vi "data_generation.vi"(0 "X Size":i32=8, 1 "slope":i16=10, 3 "scan range (um)":dbl=5.0, 4 "AmplitudeX":dbl=1.0, 5 "AmplitudeY":dbl=1.0, 6 "dwell time":i16=10, 7 "come back":i32, 8 "calibration":dbl=5.0, 9 "multicolor":dbl=5.0, 10 "zero point":dbl, 12 "first":dbl=0.5, 13 "Y size":i32=8, 15 "AmplitudeC":dbl=1.0, 17 "step size (um)":dbl=0.05, 18 "Samples per spot":i32=4, 19 "zero point 2":dbl) -> (2 "Output Graph":waveform(dbl)[](graph), 11 "DO":dbl[](array[numeric])=[0.0, 0.0, 0.0, 0.0, 0.0, 0.0, 0.0, 0.0, 1.0, 1.0, 1.0, 1.0, 1.0, 1.0, 1.0, 1.0, 2.0, 2.0, 2.0, 2.0, 2.0, 2.0, 2.0, 2.0, 3.0, 3.0, 3.0, 3.0, 3.0, 3.0, 3.0, 3.0, 4.0, 4.0, 4.0, 4.0, 4.0, 4.0, 4.0, 4.0, 5.0, 5.0, 5.0, 5.0, 5.0, 5.0, 5.0, 5.0, 6.0, 6.0, 6.0, 6.0, 6.0, 6.0, 6.0, 6.0, 7.0, 7.0, 7.0, 7.0, 7.0, 7.0, 7.0, 7.0, 7.0, 7.0, 7.0, 7.0, 7.0, 7.0, 7.0, 7.0, 6.0, 6.0, 6.0, 6.0, 6.0, 6.0, 6.0, 6.0, 5.0, 5.0, 5.0, 5.0, 5.0, 5.0, 5.0, 5.0, 4.0, 4.0, 4.0, 4.0, 4.0, 4.0, 4.0, 4.0, 3.0, 3.0, 3.0, 3.0, 3.0, 3.0, 3.0, 3.0, 2.0, 2.0, 2.0, 2.0, 2.0, 2.0, 2.0, 2.0, 1.0, 1.0, 1.0, 1.0, 1.0, 1.0, 1.0, 1.0, 0.0, 0.0, 0.0, 0.0, 0.0, 0.0, 0.0, 0.0], 14 "XY Scan":waveform(dbl)[](array[waveform])=[{"t0"=timestamp(3264022747.299 s since 1904-01-01), "dt"=0.015625, "Y"=[-1.0, -0.7142857142857143, -0.4285714285714286, -0.1428571428571429, 0.1428571428571428, 0.4285714285714286, 0.7142857142857142, 1.0, 1.0, 0.7142857142857142, 0.4285714285714286, 0.1428571428571428, -0.1428571428571429, -0.4285714285714286, -0.7142857142857143, -1.0, -1.0, -0.7142857142857143, -0.4285714285714286, -0.1428571428571429, 0.1428571428571428, 0.4285714285714286, 0.7142857142857142, 1.0, 1.0, 0.7142857142857142, 0.4285714285714286, 0.1428571428571428, -0.1428571428571429, -0.4285714285714286, -0.7142857142857143, -1.0, -1.0, -0.7142857142857143, -0.4285714285714286, -0.1428571428571429, 0.1428571428571428, 0.4285714285714286, 0.7142857142857142, 1.0, 1.0, 0.7142857142857142, 0.4285714285714286, 0.1428571428571428, -0.1428571428571429, -0.4285714285714286, -0.7142857142857143, -1.0, -1.0, -0.7142857142857143, -0.4285714285714286, -0.1428571428571429, 0.1428571428571428, 0.4285714285714286, 0.7142857142857142, 1.0, 1.0, 0.7142857142857142, 0.4285714285714286, 0.1428571428571428, -0.1428571428571429, -0.4285714285714286, -0.7142857142857143, -1.0, -1.0, -0.7142857142857143, -0.4285714285714286, -0.1428571428571429, 0.1428571428571428, 0.4285714285714286, 0.7142857142857142, 1.0, 1.0, 0.7142857142857142, 0.4285714285714286, 0.1428571428571428, -0.1428571428571429, -0.4285714285714286, -0.7142857142857143, -1.0, -1.0, -0.7142857142857143, -0.4285714285714286, -0.1428571428571429, 0.1428571428571428, 0.4285714285714286, 0.7142857142857142, 1.0, 1.0, 0.7142857142857142, 0.4285714285714286, 0.1428571428571428, -0.1428571428571429, -0.4285714285714286, -0.7142857142857143, -1.0, -1.0, -0.7142857142857143, -0.4285714285714286, -0.1428571428571429, 0.1428571428571428, 0.4285714285714286, 0.7142857142857142, 1.0, 1.0, 0.7142857142857142, 0.4285714285714286, 0.1428571428571428, -0.1428571428571429, -0.4285714285714286, -0.7142857142857143, -1.0, -1.0, -0.7142857142857143, -0.4285714285714286, -0.1428571428571429, 0.1428571428571428, 0.4285714285714286, 0.7142857142857142, 1.0, 1.0, 0.7142857142857142, 0.4285714285714286, 0.1428571428571428, -0.1428571428571429, -0.4285714285714286, -0.7142857142857143, -1.0]}, {"t0"=timestamp(3264022747.299 s since 1904-01-01), "dt"=0.015625, "Y"=[-1.0, -1.0, -1.0, -1.0, -1.0, -1.0, -1.0, -1.0, -0.7142857142857143, -0.7142857142857143, -0.7142857142857143, -0.7142857142857143, -0.7142857142857143, -0.7142857142857143, -0.7142857142857143, -0.7142857142857143, -0.4285714285714286, -0.4285714285714286, -0.4285714285714286, -0.4285714285714286, -0.4285714285714286, -0.4285714285714286, -0.4285714285714286, -0.4285714285714286, -0.1428571428571429, -0.1428571428571429, -0.1428571428571429, -0.1428571428571429, -0.1428571428571429, -0.1428571428571429, -0.1428571428571429, -0.1428571428571429, 0.1428571428571428, 0.1428571428571428, 0.1428571428571428, 0.1428571428571428, 0.1428571428571428, 0.1428571428571428, 0.1428571428571428, 0.1428571428571428, 0.4285714285714286, 0.4285714285714286, 0.4285714285714286, 0.4285714285714286, 0.4285714285714286, 0.4285714285714286, 0.4285714285714286, 0.4285714285714286, 0.7142857142857142, 0.7142857142857142, 0.7142857142857142, 0.7142857142857142, 0.7142857142857142, 0.7142857142857142, 0.7142857142857142, 0.7142857142857142, 1.0, 1.0, 1.0, 1.0, 1.0, 1.0, 1.0, 1.0, 1.0, 1.0, 1.0, 1.0, 1.0, 1.0, 1.0, 1.0, 0.7142857142857142, 0.7142857142857142, 0.7142857142857142, 0.7142857142857142, 0.7142857142857142, 0.7142857142857142, 0.7142857142857142, 0.7142857142857142, 0.4285714285714286, 0.4285714285714286, 0.4285714285714286, 0.4285714285714286, 0.4285714285714286, 0.4285714285714286, 0.4285714285714286, 0.4285714285714286, 0.1428571428571428, 0.1428571428571428, 0.1428571428571428, 0.1428571428571428, 0.1428571428571428, 0.1428571428571428, 0.1428571428571428, 0.1428571428571428, -0.1428571428571429, -0.1428571428571429, -0.1428571428571429, -0.1428571428571429, -0.1428571428571429, -0.1428571428571429, -0.1428571428571429, -0.1428571428571429, -0.4285714285714286, -0.4285714285714286, -0.4285714285714286, -0.4285714285714286, -0.4285714285714286, -0.4285714285714286, -0.4285714285714286, -0.4285714285714286, -0.7142857142857143, -0.7142857142857143, -0.7142857142857143, -0.7142857142857143, -0.7142857142857143, -0.7142857142857143, -0.7142857142857143, -0.7142857142857143, -1.0, -1.0, -1.0, -1.0, -1.0, -1.0, -1.0, -1.0]}])   [LabVIEW 2017]
uses:
  Instance           2 16Saved   scan_1_5 .vi
  Instance           3 16Saved   scan_1_5 .vi
  <vilib>/Analysis/3filter.llb/Zero Phase Filter (DBL).vi
  <vilib>/Analysis/NI_AALBase.lvlib
panel:
  out "AO Data":dbl[][](array[numeric])
  out "nanoZ output":dbl[](array[numeric])=[-1.0, -1.0, -1.0, -1.0, -1.0, -1.0, -1.0, -1.0, -0.7142857142857143, -0.7142857142857143, -0.7142857142857143, -0.7142857142857143, -0.7142857142857143, -0.7142857142857143, -0.7142857142857143, -0.7142857142857143, -0.4285714285714286, -0.4285714285714286, -0.4285714285714286, -0.4285714285714286, -0.4285714285714286, -0.4285714285714286, -0.4285714285714286, -0.4285714285714286, -0.1428571428571429, -0.1428571428571429, -0.1428571428571429, -0.1428571428571429, -0.1428571428571429, -0.1428571428571429, -0.1428571428571429, -0.1428571428571429, 0.1428571428571428, 0.1428571428571428, 0.1428571428571428, 0.1428571428571428, 0.1428571428571428, 0.1428571428571428, 0.1428571428571428, 0.1428571428571428, 0.4285714285714286, 0.4285714285714286, 0.4285714285714286, 0.4285714285714286, 0.4285714285714286, 0.4285714285714286, 0.4285714285714286, 0.4285714285714286, 0.7142857142857142, 0.7142857142857142, 0.7142857142857142, 0.7142857142857142, 0.7142857142857142, 0.7142857142857142, 0.7142857142857142, 0.7142857142857142, 1.0, 1.0, 1.0, 1.0, 1.0, 1.0, 1.0, 1.0, 1.0, 1.0, 1.0, 1.0, 1.0, 1.0, 1.0, 1.0, 0.7142857142857142, 0.7142857142857142, 0.7142857142857142, 0.7142857142857142, 0.7142857142857142, 0.7142857142857142, 0.7142857142857142, 0.7142857142857142, 0.4285714285714286, 0.4285714285714286, 0.4285714285714286, 0.4285714285714286, 0.4285714285714286, 0.4285714285714286, 0.4285714285714286, 0.4285714285714286, 0.1428571428571428, 0.1428571428571428, 0.1428571428571428, 0.1428571428571428, 0.1428571428571428, 0.1428571428571428, 0.1428571428571428, 0.1428571428571428, -0.1428571428571429, -0.1428571428571429, -0.1428571428571429, -0.1428571428571429, -0.1428571428571429, -0.1428571428571429, -0.1428571428571429, -0.1428571428571429, -0.4285714285714286, -0.4285714285714286, -0.4285714285714286, -0.4285714285714286, -0.4285714285714286, -0.4285714285714286, -0.4285714285714286, -0.4285714285714286, -0.7142857142857143, -0.7142857142857143, -0.7142857142857143, -0.7142857142857143, -0.7142857142857143, -0.7142857142857143, -0.7142857142857143, -0.7142857142857143, -1.0, -1.0, -1.0, -1.0, -1.0, -1.0, -1.0, -1.0]
  out "nanoZ":dbl[](array[numeric])=[0.0, 1.0, 2.0, 3.0, 4.0, 5.0, 6.0, 7.0, 7.0, 6.0, 5.0, 4.0, 3.0, 2.0, 1.0, 0.0, 0.0, 1.0, 2.0, 3.0, 4.0, 5.0, 6.0, 7.0, 7.0, 6.0, 5.0, 4.0, 3.0, 2.0, 1.0, 0.0, 0.0, 1.0, 2.0, 3.0, 4.0, 5.0, 6.0, 7.0, 7.0, 6.0, 5.0, 4.0, 3.0, 2.0, 1.0, 0.0, 0.0, 1.0, 2.0, 3.0, 4.0, 5.0, 6.0, 7.0, 7.0, 6.0, 5.0, 4.0, 3.0, 2.0, 1.0, 0.0, 0.0, 1.0, 2.0, 3.0, 4.0, 5.0, 6.0, 7.0, 7.0, 6.0, 5.0, 4.0, 3.0, 2.0, 1.0, 0.0, 0.0, 1.0, 2.0, 3.0, 4.0, 5.0, 6.0, 7.0, 7.0, 6.0, 5.0, 4.0, 3.0, 2.0, 1.0, 0.0, 0.0, 1.0, 2.0, 3.0, 4.0, 5.0, 6.0, 7.0, 7.0, 6.0, 5.0, 4.0, 3.0, 2.0, 1.0, 0.0, 0.0, 1.0, 2.0, 3.0, 4.0, 5.0, 6.0, 7.0, 7.0, 6.0, 5.0, 4.0, 3.0, 2.0, 1.0, 0.0]
  out "Trigger output":dbl[](array[numeric])=[-1.0, -1.0, -1.0, -1.0, -1.0, -1.0, -1.0, -1.0, -0.7142857142857143, -0.7142857142857143, -0.7142857142857143, -0.7142857142857143, -0.7142857142857143, -0.7142857142857143, -0.7142857142857143, -0.7142857142857143, -0.4285714285714286, -0.4285714285714286, -0.4285714285714286, -0.4285714285714286, -0.4285714285714286, -0.4285714285714286, -0.4285714285714286, -0.4285714285714286, -0.1428571428571429, -0.1428571428571429, -0.1428571428571429, -0.1428571428571429, -0.1428571428571429, -0.1428571428571429, -0.1428571428571429, -0.1428571428571429, 0.1428571428571428, 0.1428571428571428, 0.1428571428571428, 0.1428571428571428, 0.1428571428571428, 0.1428571428571428, 0.1428571428571428, 0.1428571428571428, 0.4285714285714286, 0.4285714285714286, 0.4285714285714286, 0.4285714285714286, 0.4285714285714286, 0.4285714285714286, 0.4285714285714286, 0.4285714285714286, 0.7142857142857142, 0.7142857142857142, 0.7142857142857142, 0.7142857142857142, 0.7142857142857142, 0.7142857142857142, 0.7142857142857142, 0.7142857142857142, 1.0, 1.0, 1.0, 1.0, 1.0, 1.0, 1.0, 1.0, 1.0, 1.0, 1.0, 1.0, 1.0, 1.0, 1.0, 1.0, 0.7142857142857142, 0.7142857142857142, 0.7142857142857142, 0.7142857142857142, 0.7142857142857142, 0.7142857142857142, 0.7142857142857142, 0.7142857142857142, 0.4285714285714286, 0.4285714285714286, 0.4285714285714286, 0.4285714285714286, 0.4285714285714286, 0.4285714285714286, 0.4285714285714286, 0.4285714285714286, 0.1428571428571428, 0.1428571428571428, 0.1428571428571428, 0.1428571428571428, 0.1428571428571428, 0.1428571428571428, 0.1428571428571428, 0.1428571428571428, -0.1428571428571429, -0.1428571428571429, -0.1428571428571429, -0.1428571428571429, -0.1428571428571429, -0.1428571428571429, -0.1428571428571429, -0.1428571428571429, -0.4285714285714286, -0.4285714285714286, -0.4285714285714286, -0.4285714285714286, -0.4285714285714286, -0.4285714285714286, -0.4285714285714286, -0.4285714285714286, -0.7142857142857143, -0.7142857142857143, -0.7142857142857143, -0.7142857142857143, -0.7142857142857143, -0.7142857142857143, -0.7142857142857143, -0.7142857142857143, -1.0, -1.0, -1.0, -1.0, -1.0, -1.0, -1.0, -1.0]
  out "Trigger":dbl[](array[numeric])=[0.0, 0.0, 0.0, 0.0, 0.0, 0.0, 0.0, 0.0, 1.0, 1.0, 1.0, 1.0, 1.0, 1.0, 1.0, 1.0, 2.0, 2.0, 2.0, 2.0, 2.0, 2.0, 2.0, 2.0, 3.0, 3.0, 3.0, 3.0, 3.0, 3.0, 3.0, 3.0, 4.0, 4.0, 4.0, 4.0, 4.0, 4.0, 4.0, 4.0, 5.0, 5.0, 5.0, 5.0, 5.0, 5.0, 5.0, 5.0, 6.0, 6.0, 6.0, 6.0, 6.0, 6.0, 6.0, 6.0, 7.0, 7.0, 7.0, 7.0, 7.0, 7.0, 7.0, 7.0, 7.0, 7.0, 7.0, 7.0, 7.0, 7.0, 7.0, 7.0, 6.0, 6.0, 6.0, 6.0, 6.0, 6.0, 6.0, 6.0, 5.0, 5.0, 5.0, 5.0, 5.0, 5.0, 5.0, 5.0, 4.0, 4.0, 4.0, 4.0, 4.0, 4.0, 4.0, 4.0, 3.0, 3.0, 3.0, 3.0, 3.0, 3.0, 3.0, 3.0, 2.0, 2.0, 2.0, 2.0, 2.0, 2.0, 2.0, 2.0, 1.0, 1.0, 1.0, 1.0, 1.0, 1.0, 1.0, 1.0, 0.0, 0.0, 0.0, 0.0, 0.0, 0.0, 0.0, 0.0]
  out "Waveform Graph":dynamicdata(graph)
  in  "dt":dbl=1e-05
  out "time":dbl=3264022747.299 format="%<%I:%M:%S %p\n%m/%d/%Y>T"
  out "Y output Array":dbl[](array[numeric])=[-1.0, -1.0, -1.0, -1.0, -1.0, -1.0, -1.0, -1.0, -0.7142857142857143, -0.7142857142857143, -0.7142857142857143, -0.7142857142857143, -0.7142857142857143, -0.7142857142857143, -0.7142857142857143, -0.7142857142857143, -0.4285714285714286, -0.4285714285714286, -0.4285714285714286, -0.4285714285714286, -0.4285714285714286, -0.4285714285714286, -0.4285714285714286, -0.4285714285714286, -0.1428571428571429, -0.1428571428571429, -0.1428571428571429, -0.1428571428571429, -0.1428571428571429, -0.1428571428571429, -0.1428571428571429, -0.1428571428571429, 0.1428571428571428, 0.1428571428571428, 0.1428571428571428, 0.1428571428571428, 0.1428571428571428, 0.1428571428571428, 0.1428571428571428, 0.1428571428571428, 0.4285714285714286, 0.4285714285714286, 0.4285714285714286, 0.4285714285714286, 0.4285714285714286, 0.4285714285714286, 0.4285714285714286, 0.4285714285714286, 0.7142857142857142, 0.7142857142857142, 0.7142857142857142, 0.7142857142857142, 0.7142857142857142, 0.7142857142857142, 0.7142857142857142, 0.7142857142857142, 1.0, 1.0, 1.0, 1.0, 1.0, 1.0, 1.0, 1.0, 1.0, 1.0, 1.0, 1.0, 1.0, 1.0, 1.0, 1.0, 0.7142857142857142, 0.7142857142857142, 0.7142857142857142, 0.7142857142857142, 0.7142857142857142, 0.7142857142857142, 0.7142857142857142, 0.7142857142857142, 0.4285714285714286, 0.4285714285714286, 0.4285714285714286, 0.4285714285714286, 0.4285714285714286, 0.4285714285714286, 0.4285714285714286, 0.4285714285714286, 0.1428571428571428, 0.1428571428571428, 0.1428571428571428, 0.1428571428571428, 0.1428571428571428, 0.1428571428571428, 0.1428571428571428, 0.1428571428571428, -0.1428571428571429, -0.1428571428571429, -0.1428571428571429, -0.1428571428571429, -0.1428571428571429, -0.1428571428571429, -0.1428571428571429, -0.1428571428571429, -0.4285714285714286, -0.4285714285714286, -0.4285714285714286, -0.4285714285714286, -0.4285714285714286, -0.4285714285714286, -0.4285714285714286, -0.4285714285714286, -0.7142857142857143, -0.7142857142857143, -0.7142857142857143, -0.7142857142857143, -0.7142857142857143, -0.7142857142857143, -0.7142857142857143, -0.7142857142857143, -1.0, -1.0, -1.0, -1.0, -1.0, -1.0, -1.0, -1.0]
  out "X output Array":dbl[](array[numeric])=[-1.0, -0.7142857142857143, -0.4285714285714286, -0.1428571428571429, 0.1428571428571428, 0.4285714285714286, 0.7142857142857142, 1.0, 1.0, 0.7142857142857142, 0.4285714285714286, 0.1428571428571428, -0.1428571428571429, -0.4285714285714286, -0.7142857142857143, -1.0, -1.0, -0.7142857142857143, -0.4285714285714286, -0.1428571428571429, 0.1428571428571428, 0.4285714285714286, 0.7142857142857142, 1.0, 1.0, 0.7142857142857142, 0.4285714285714286, 0.1428571428571428, -0.1428571428571429, -0.4285714285714286, -0.7142857142857143, -1.0, -1.0, -0.7142857142857143, -0.4285714285714286, -0.1428571428571429, 0.1428571428571428, 0.4285714285714286, 0.7142857142857142, 1.0, 1.0, 0.7142857142857142, 0.4285714285714286, 0.1428571428571428, -0.1428571428571429, -0.4285714285714286, -0.7142857142857143, -1.0, -1.0, -0.7142857142857143, -0.4285714285714286, -0.1428571428571429, 0.1428571428571428, 0.4285714285714286, 0.7142857142857142, 1.0, 1.0, 0.7142857142857142, 0.4285714285714286, 0.1428571428571428, -0.1428571428571429, -0.4285714285714286, -0.7142857142857143, -1.0, -1.0, -0.7142857142857143, -0.4285714285714286, -0.1428571428571429, 0.1428571428571428, 0.4285714285714286, 0.7142857142857142, 1.0, 1.0, 0.7142857142857142, 0.4285714285714286, 0.1428571428571428, -0.1428571428571429, -0.4285714285714286, -0.7142857142857143, -1.0, -1.0, -0.7142857142857143, -0.4285714285714286, -0.1428571428571429, 0.1428571428571428, 0.4285714285714286, 0.7142857142857142, 1.0, 1.0, 0.7142857142857142, 0.4285714285714286, 0.1428571428571428, -0.1428571428571429, -0.4285714285714286, -0.7142857142857143, -1.0, -1.0, -0.7142857142857143, -0.4285714285714286, -0.1428571428571429, 0.1428571428571428, 0.4285714285714286, 0.7142857142857142, 1.0, 1.0, 0.7142857142857142, 0.4285714285714286, 0.1428571428571428, -0.1428571428571429, -0.4285714285714286, -0.7142857142857143, -1.0, -1.0, -0.7142857142857143, -0.4285714285714286, -0.1428571428571429, 0.1428571428571428, 0.4285714285714286, 0.7142857142857142, 1.0, 1.0, 0.7142857142857142, 0.4285714285714286, 0.1428571428571428, -0.1428571428571429, -0.4285714285714286, -0.7142857142857143, -1.0]
  out "Y index Array":dbl[](array[numeric])=[0.0, 0.0, 0.0, 0.0, 0.0, 0.0, 0.0, 0.0, 1.0, 1.0, 1.0, 1.0, 1.0, 1.0, 1.0, 1.0, 2.0, 2.0, 2.0, 2.0, 2.0, 2.0, 2.0, 2.0, 3.0, 3.0, 3.0, 3.0, 3.0, 3.0, 3.0, 3.0, 4.0, 4.0, 4.0, 4.0, 4.0, 4.0, 4.0, 4.0, 5.0, 5.0, 5.0, 5.0, 5.0, 5.0, 5.0, 5.0, 6.0, 6.0, 6.0, 6.0, 6.0, 6.0, 6.0, 6.0, 7.0, 7.0, 7.0, 7.0, 7.0, 7.0, 7.0, 7.0, 7.0, 7.0, 7.0, 7.0, 7.0, 7.0, 7.0, 7.0, 6.0, 6.0, 6.0, 6.0, 6.0, 6.0, 6.0, 6.0, 5.0, 5.0, 5.0, 5.0, 5.0, 5.0, 5.0, 5.0, 4.0, 4.0, 4.0, 4.0, 4.0, 4.0, 4.0, 4.0, 3.0, 3.0, 3.0, 3.0, 3.0, 3.0, 3.0, 3.0, 2.0, 2.0, 2.0, 2.0, 2.0, 2.0, 2.0, 2.0, 1.0, 1.0, 1.0, 1.0, 1.0, 1.0, 1.0, 1.0, 0.0, 0.0, 0.0, 0.0, 0.0, 0.0, 0.0, 0.0]
  out "X index Array":dbl[](array[numeric])=[0.0, 1.0, 2.0, 3.0, 4.0, 5.0, 6.0, 7.0, 7.0, 6.0, 5.0, 4.0, 3.0, 2.0, 1.0, 0.0, 0.0, 1.0, 2.0, 3.0, 4.0, 5.0, 6.0, 7.0, 7.0, 6.0, 5.0, 4.0, 3.0, 2.0, 1.0, 0.0, 0.0, 1.0, 2.0, 3.0, 4.0, 5.0, 6.0, 7.0, 7.0, 6.0, 5.0, 4.0, 3.0, 2.0, 1.0, 0.0, 0.0, 1.0, 2.0, 3.0, 4.0, 5.0, 6.0, 7.0, 7.0, 6.0, 5.0, 4.0, 3.0, 2.0, 1.0, 0.0, 0.0, 1.0, 2.0, 3.0, 4.0, 5.0, 6.0, 7.0, 7.0, 6.0, 5.0, 4.0, 3.0, 2.0, 1.0, 0.0, 0.0, 1.0, 2.0, 3.0, 4.0, 5.0, 6.0, 7.0, 7.0, 6.0, 5.0, 4.0, 3.0, 2.0, 1.0, 0.0, 0.0, 1.0, 2.0, 3.0, 4.0, 5.0, 6.0, 7.0, 7.0, 6.0, 5.0, 4.0, 3.0, 2.0, 1.0, 0.0, 0.0, 1.0, 2.0, 3.0, 4.0, 5.0, 6.0, 7.0, 7.0, 6.0, 5.0, 4.0, 3.0, 2.0, 1.0, 0.0]
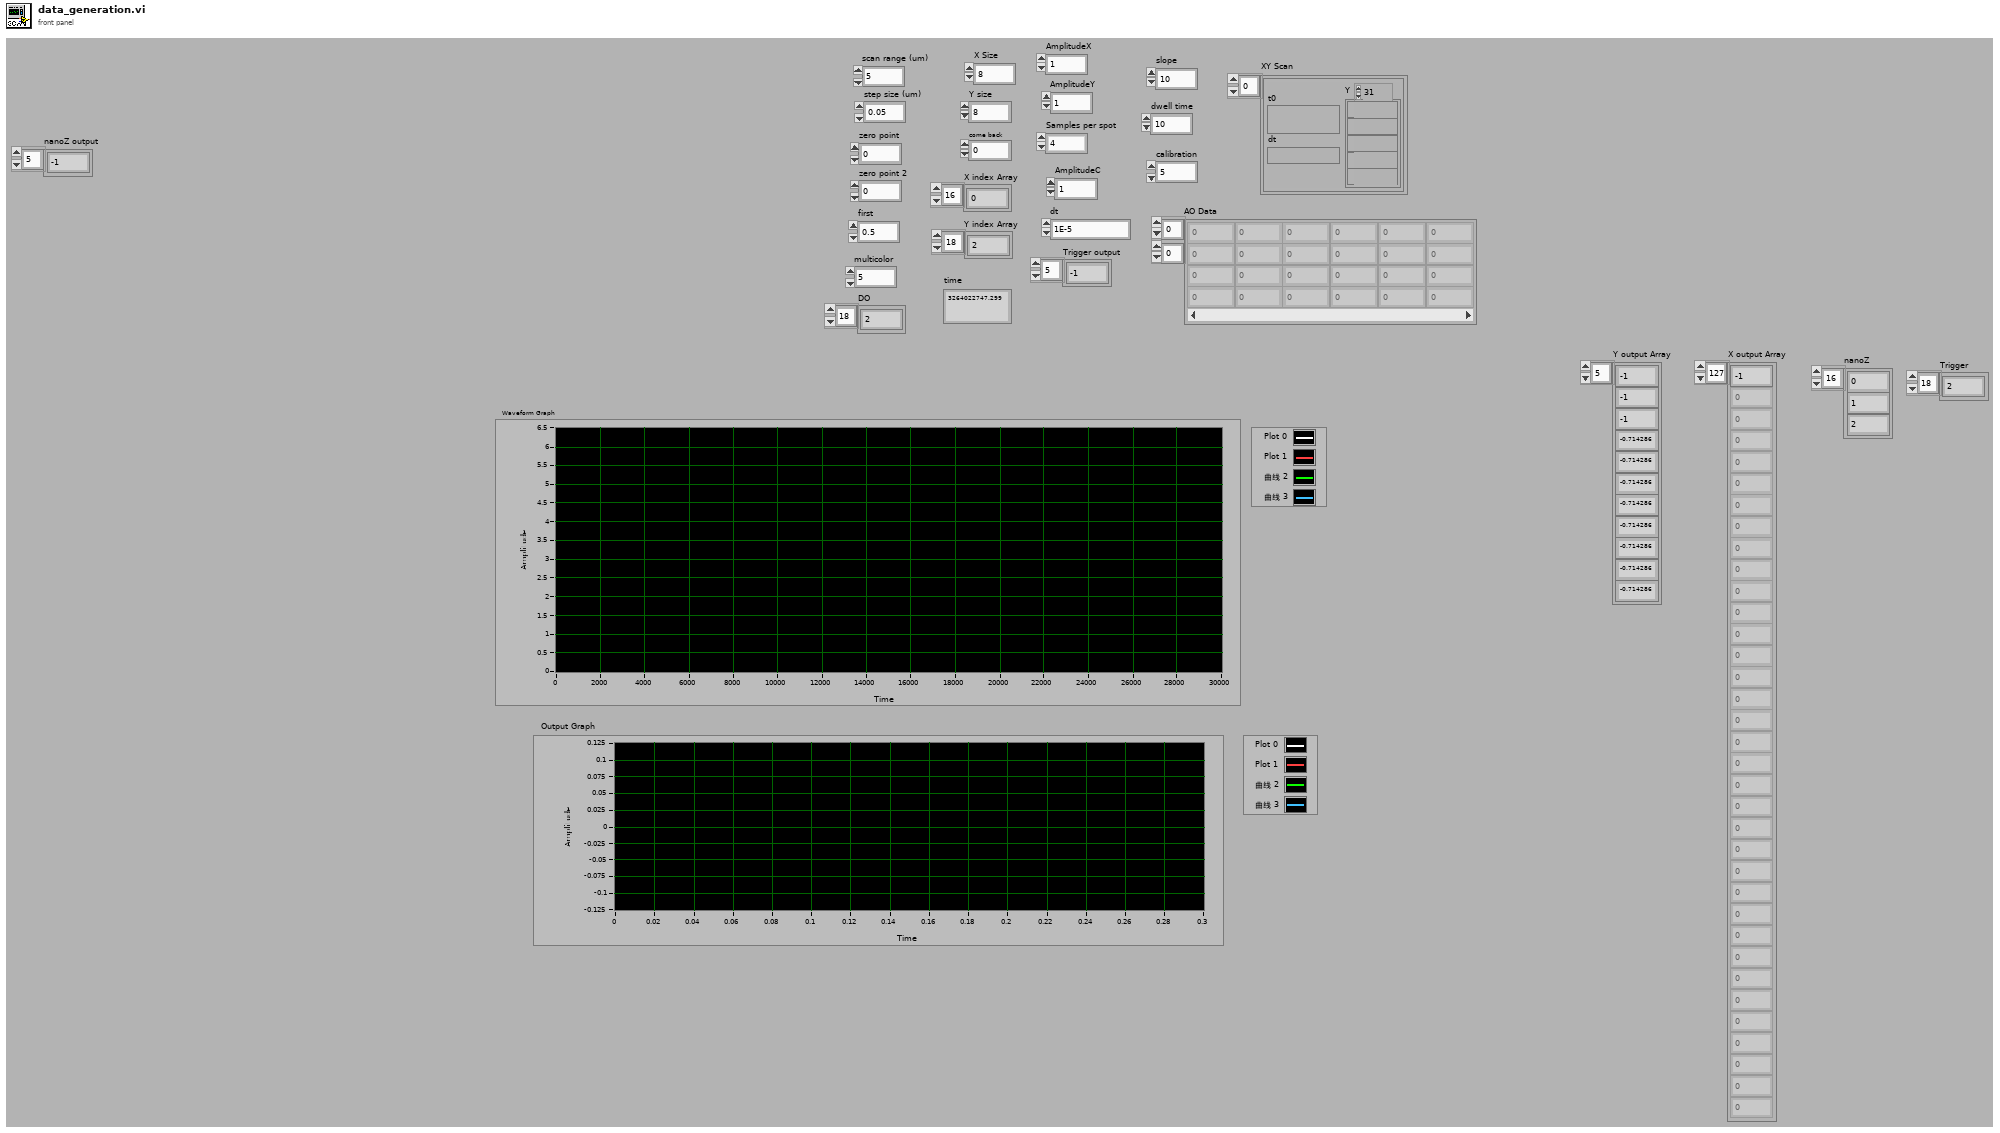
[diagram p1: front panel]
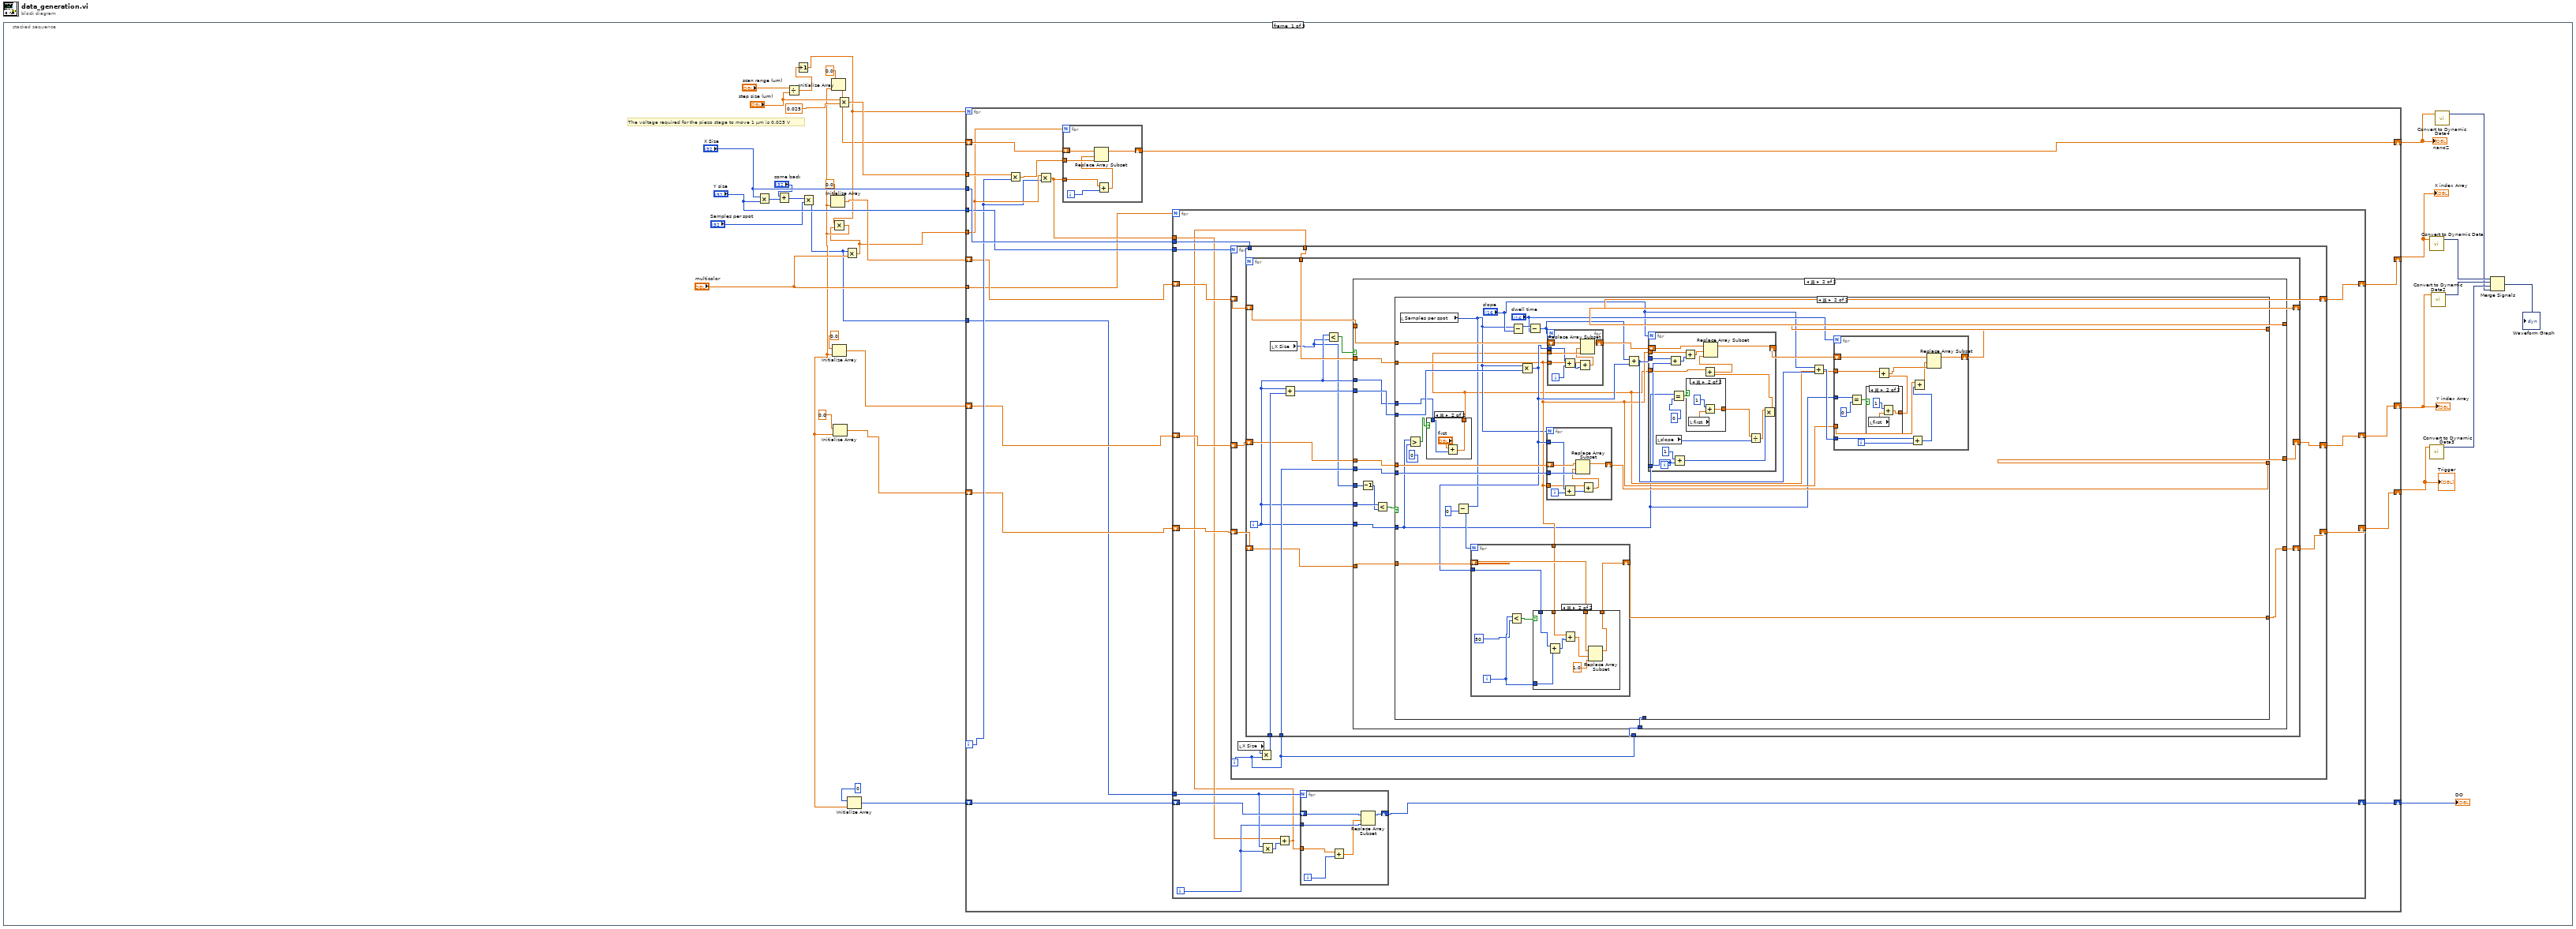
[diagram p0: block diagram]
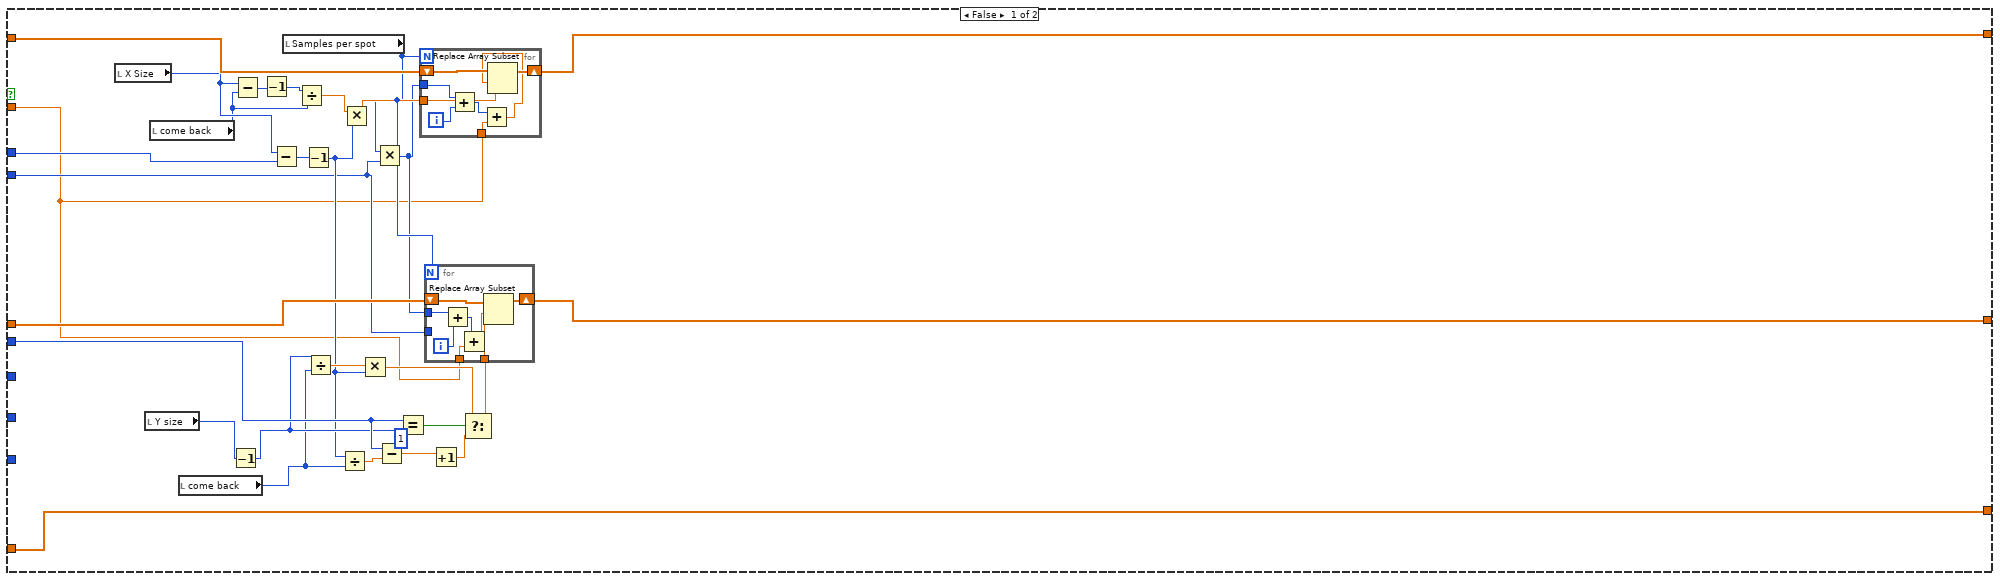
[diagram p2: hidden frame]
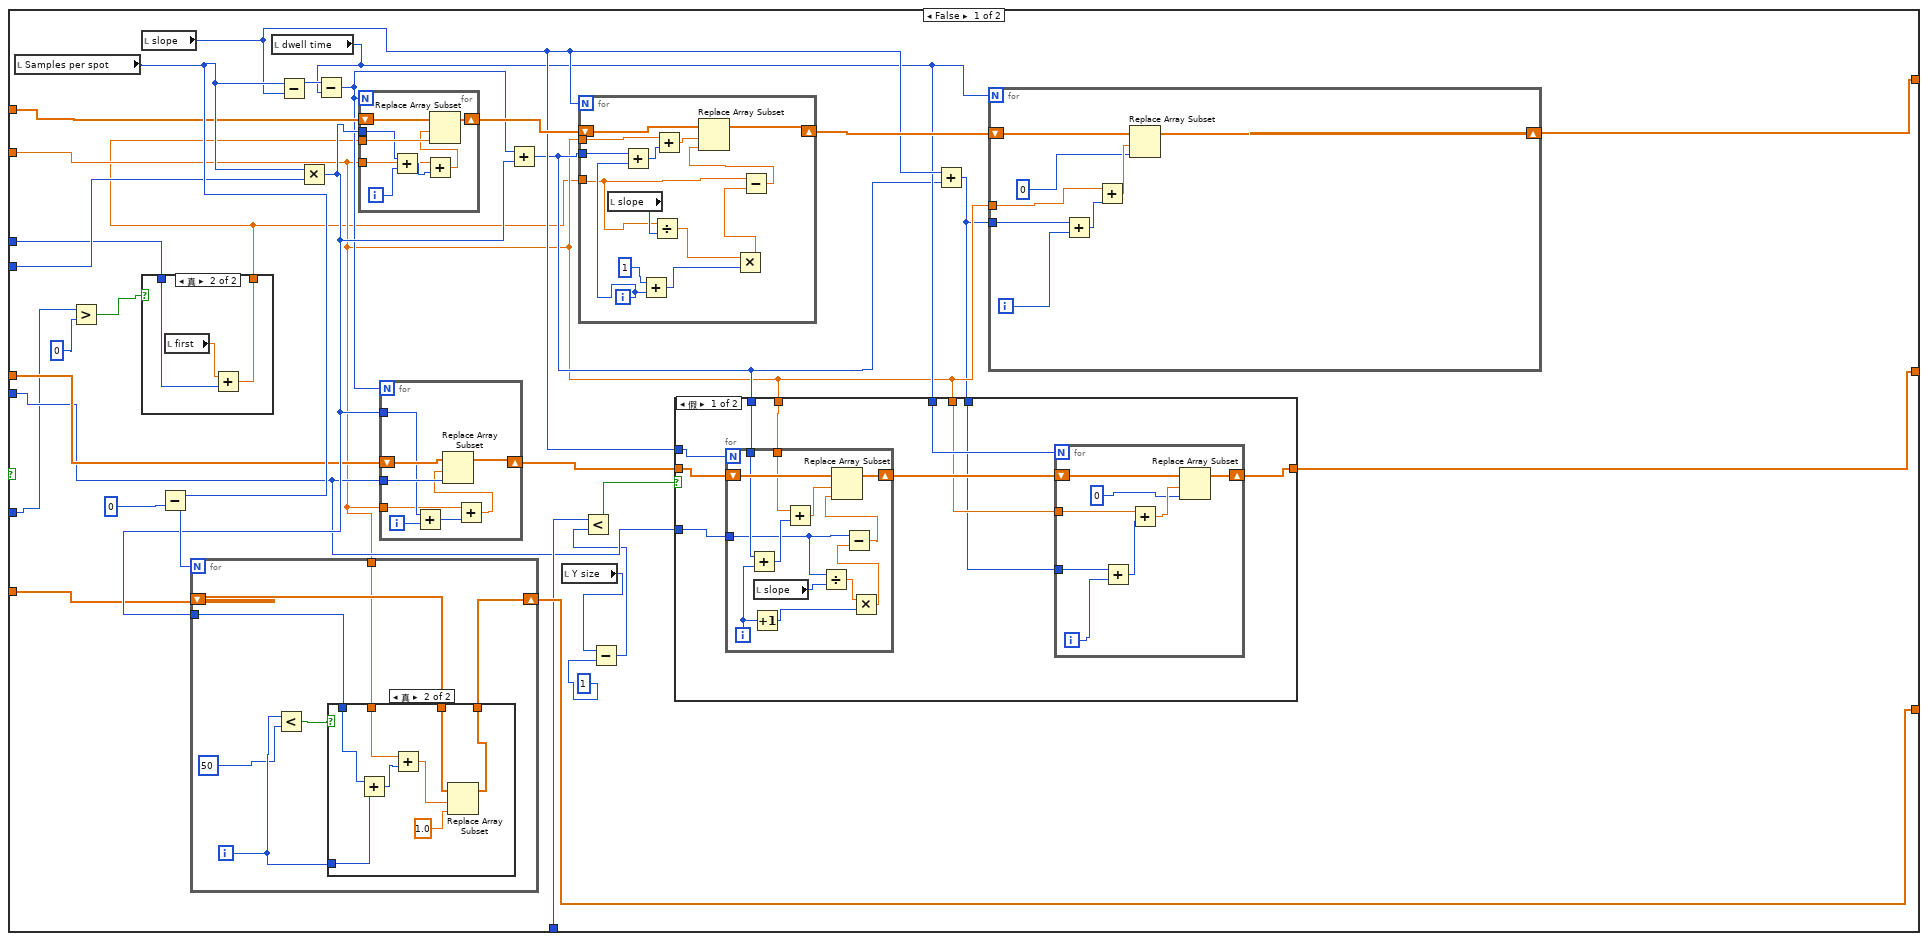
[diagram p3: hidden frame]
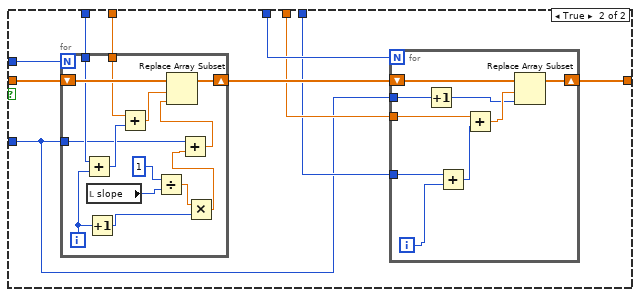
[diagram p5: hidden frame]
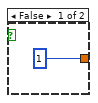
[diagram p8: hidden frame]
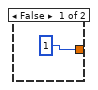
[diagram p9: hidden frame]
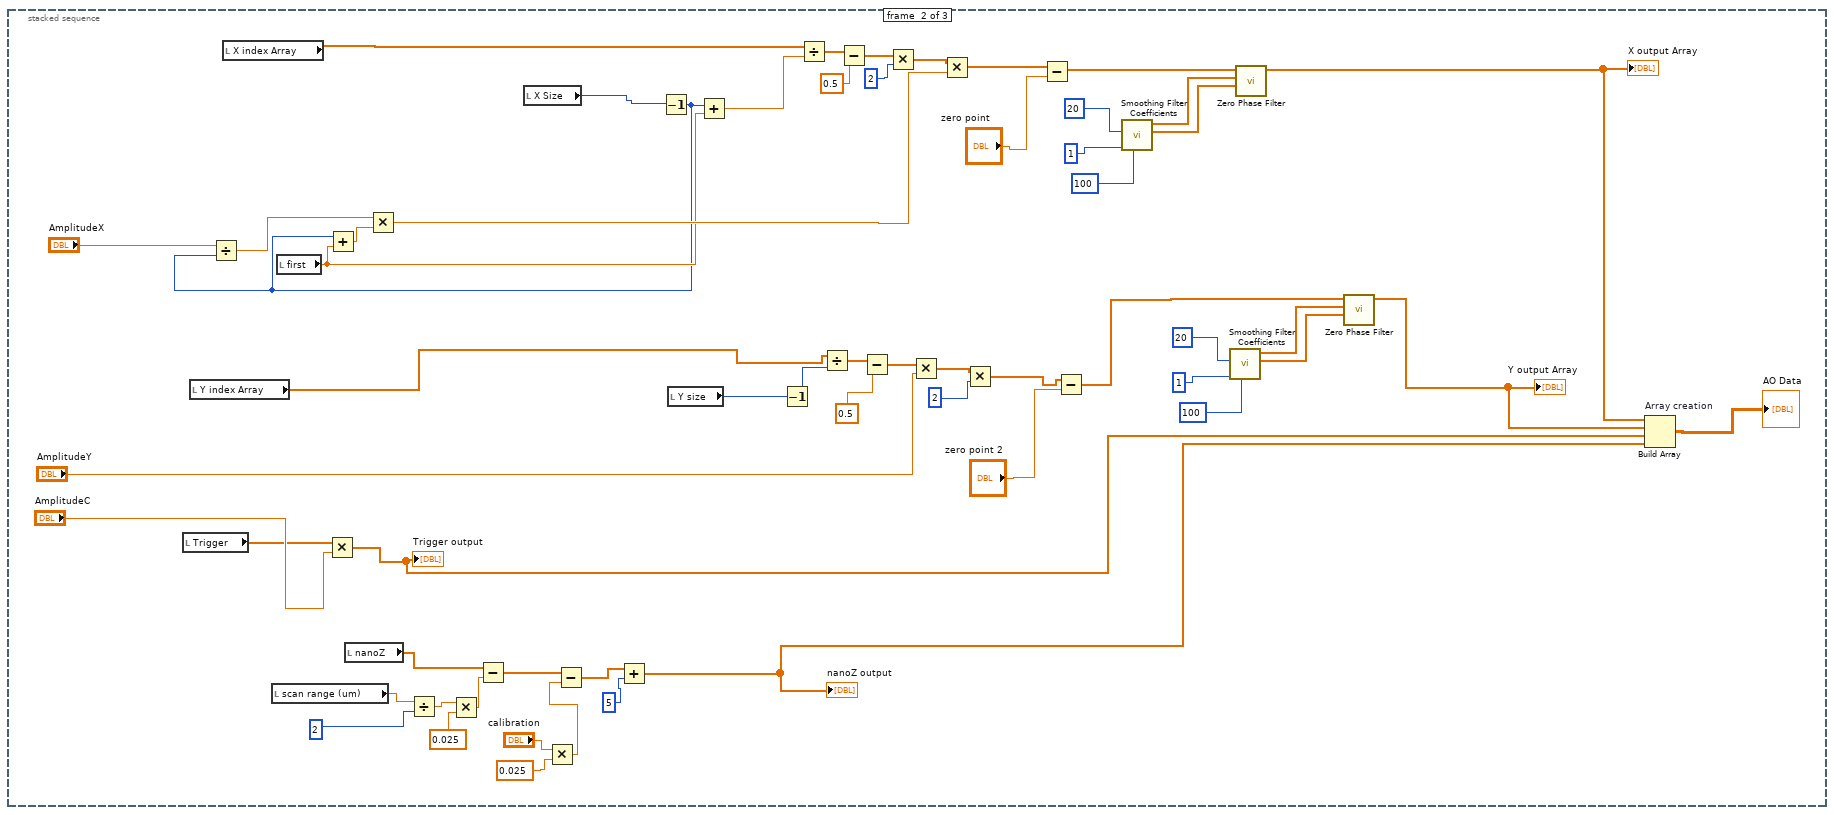
[diagram p11: hidden frame]
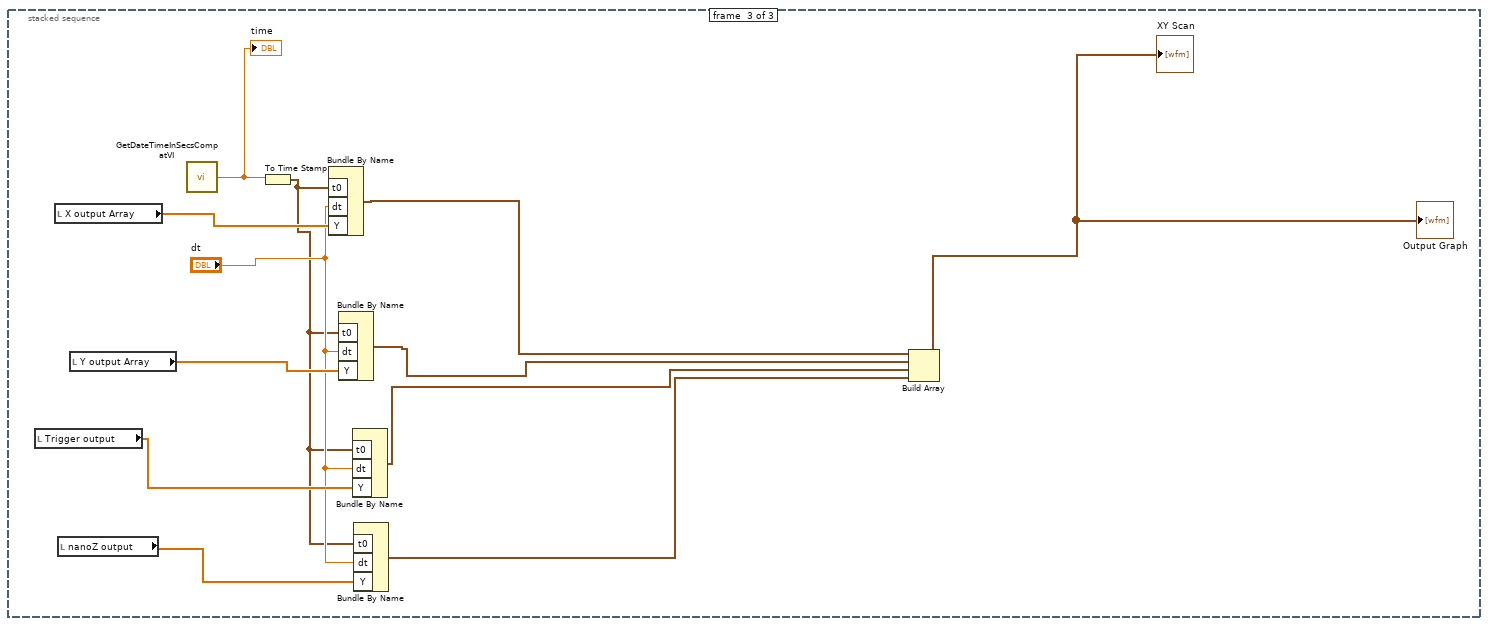
[diagram p12: hidden frame]
diagram:
  n1 = stacked-sequence {
    frame #0 {
      # "The voltage required for the piezo stage to move 1 μm is 0.025 V"
      n2 = Multiply(x="X Size", y="Y size") -> (x*y=w9:i32)
      n3 = Add(x="come back", y=w9) -> (x+y=w8:i32)
      n4 = Divide(x="scan range (um)", y="step size (um)") -> (x/y=w16:dbl)
      n5 = Increment(x=w16) -> (x+1=w17:dbl)
      n6 = Multiply(x=w8, y="Samples per spot") -> (x*y=w1:i32)
      n7 = Multiply(x="step size (um)", y=0.025) -> (x*y=w21:dbl)
      n8 = Multiply(x=w1, y="multicolor") -> (x*y=w2:dbl)
      n9 = Multiply(x=w17, y=w2) -> (x*y=w3:dbl)
      n10 = Initialize Array(0.0, w3) -> (w24:dbl[])
      n11 = Initialize Array(0.0, w3) -> (w11:dbl[])
      n12 = Initialize Array(0.0, w3) -> (w25:dbl[])
      n13 = Initialize Array(0.0, w3) -> (w26:dbl[])
      n14 = Initialize Array(0, w3) -> (w6:i32[])
      n15 = for {
        N: w17 -> [_]
        tunnel: "X Size" -> [w53]
        tunnel: "Y size" -> [w52]
        shift-right: [w55] -> w13
        shift-left: w25 -> [w43]
        shift-right: [w42] -> w12
        shift-left: w26 -> [w41]
        shift-right: [w54] -> w14
        shift-left: w24 -> [w44]
        tunnel: w21 -> [w51]
        tunnel: w2 -> [w47]
        shift-right: [w48] -> w15
        shift-left: w11 -> [w50]
        tunnel: "multicolor" -> [w40]
        shift-right: [w38] -> w5
        shift-left: w6 -> [w39]
        tunnel: w1 -> [w37]
        i -> [w46]
        n16 = Multiply(x=w51, y=w46) -> (x*y=w49:dbl)
        n17 = Multiply(x=w47, y=w46) -> (x*y=w45:dbl)
        n18 = for {
          N: w47 -> [_]
          shift-right: [w422] -> w48
          shift-left: w50 -> [w423]
          tunnel: w49 -> [w421]
          tunnel: w45 -> [w418]
          i -> [w420]
          n19 = Add(x=w418, y=w420) -> (x+y=w419:dbl)
          n20 = Replace Array Subset(array=w423, new element=w421, index=w419) -> (w422:dbl[])
        }
        n21 = for {
          N: w40 -> [_]
          tunnel: w53 -> [w68]
          tunnel: w52 -> [w67]
          tunnel: w45 -> [w57]
          shift-right: [w69] -> w54
          shift-left: w44 -> [w66]
          shift-right: [w70] -> w55
          shift-left: w43 -> [w65]
          shift-right: [w64] -> w42
          shift-left: w41 -> [w63]
          shift-right: [w61] -> w38
          shift-left: w39 -> [w62]
          tunnel: w37 -> [w60]
          i -> [w59]
          n22 = Multiply(x=w60, y=w59) -> (x*y=w58:i32)
          n23 = Add(x=w57, y=w58) -> (x+y=w56:dbl)
          n24 = for {
            N: w67 -> [_]
            tunnel: w68 -> [w87]
            shift-right: [w85] -> w69
            shift-left: w66 -> [w86]
            shift-right: [w81] -> w70
            shift-left: w65 -> [w82]
            shift-right: [w79] -> w64
            shift-left: w63 -> [w80]
            tunnel: w56 -> [w78]
            i -> [w77]
            n25 = local read "X Size"() -> (w84:i32)
            n26 = Multiply(x=w84, y=w77) -> (x*y=w83:i32)
            n27 = for {
              N: w87 -> [_]
              shift-right: [w100] -> w85
              shift-left: w86 -> [w101]
              tunnel: w83 -> [w99]
              shift-right: [w95] -> w81
              shift-left: w82 -> [w96]
              tunnel: w77 -> [w94]
              shift-right: [w88] -> w79
              shift-left: w80 -> [w93]
              tunnel: w78 -> [w92]
              tunnel: w77 -> [w91]
              i -> [w90]
              n28 = local read "X Size"() -> (w89:i32)
              n29 = Add(x=w90, y=w99) -> (x+y=w98:i32)
              n30 = Less?(x=w90, y=w89) -> (x < y?=w97:bool)
              n31 = case shown="真" w97 {
                tunnel: w101 -> [w130 w162]
                tunnel: [w129 w156] -> w100
                tunnel: w98 -> [w108 w158]
                tunnel: w90 -> [w124 w155]
                tunnel: w96 -> [w120 w161]
                tunnel: [w119 w160] -> w95
                tunnel: w94 -> [w116 w159]
                tunnel: w93 -> [w102 w157]
                tunnel: w90 -> [_ w154]
                tunnel: w89 -> [_ w152]
                tunnel: w92 -> [w103 w150]
                tunnel: w91 -> [_ w149]
                tunnel: w90 -> [_ w148]
                tunnel: [w102 w147] -> w88
                frame False {
                  (unwired) 1
                  n32 = local read "X Size"() -> (w123:i32)
                  n33 = local read "Y size"() -> (w104:i32)
                  n34 = local read "come back"() -> (w121:i32)
                  n35 = local read "come back"() -> (w105:i32)
                  n36 = Decrement(x=w104) -> (x-1=w112:i32)
                  n37 = Subtract(x=w123, y=w121) -> (x-y=w128:i32)
                  n38 = Decrement(x=w128) -> (x-1=w127:i32)
                  n39 = Subtract(x=w123, y=w124) -> (x-y=w125:i32)
                  n40 = local read "Samples per spot"() -> (w107:i32)
                  n41 = Divide(x=w127, y=w121) -> (x/y=w126:dbl)
                  n42 = Decrement(x=w125) -> (x-1=w110:i32)
                  n43 = Divide(x=w112, y=w105) -> (x/y=w111:dbl)
                  n44 = Divide(x=w110, y=w105) -> (x/y=w117:dbl)
                  n45 = Multiply(x=w126, y=w110) -> (x*y=w122:dbl)
                  n46 = Multiply(x=w111, y=w110) -> (x*y=w109:dbl)
                  n47 = Multiply(x=w107, y=w108) -> (x*y=w106:i32)
                  n48 = Subtract(x=w116, y=w117) -> (x-y=w114:dbl)
                  n49 = Equal?(x=w116, y=w112) -> (x = y?=w118:bool)
                  n50 = for {
                    N: w107 -> [_]
                    tunnel: w122 -> [w144]
                    shift-right: [w145] -> w129
                    shift-left: w130 -> [w146]
                    tunnel: w106 -> [w142]
                    tunnel: w103 -> [w139]
                    i -> [w143]
                    n51 = Add(x=w142, y=w143) -> (x+y=w141:i32)
                    n52 = Add(x=w141, y=w139) -> (x+y=w140:dbl)
                    n53 = Replace Array Subset(array=w146, new element=w144, index=w140) -> (w145:dbl[])
                  }
                  n54 = Increment(x=w114) -> (x+1=w113:dbl)
                  n55 = Select(t=w109, s=w118, f=w113) -> (s? t:f=w115:dbl)
                  n56 = for {
                    N: w107 -> [_]
                    tunnel: w108 -> [_]
                    tunnel: w115 -> [w136]
                    shift-right: [w137] -> w119
                    shift-left: w120 -> [w138]
                    tunnel: w106 -> [w135]
                    tunnel: w103 -> [w131]
                    i -> [w134]
                    n57 = Add(x=w135, y=w134) -> (x+y=w133:i32)
                    n58 = Add(x=w133, y=w131) -> (x+y=w132:dbl)
                    n59 = Replace Array Subset(array=w138, new element=w136, index=w132) -> (w137:dbl[])
                  }
                }
                frame True {
                  n60 = Decrement(x=w152) -> (x-1=w153:i32)
                  n61 = Less?(x=w154, y=w153) -> (x < y?=w151:bool)
                  n62 = case shown="真" w151 {
                    tunnel: w162 -> [w187 w342]
                    tunnel: w161 -> [w185 w341]
                    tunnel: [w166 w340] -> w160
                    tunnel: w159 -> [w176 w339]
                    tunnel: w158 -> [w186 w338]
                    tunnel: w157 -> [w184 w337]
                    tunnel: [w183 w334] -> w147
                    tunnel: [w167 w330] -> w156
                    tunnel: w155 -> [w172 w320]
                    tunnel: w150 -> [w175 w323]
                    tunnel: w149 -> [w182 _]
                    tunnel: w148 -> [w170 w319]
                    frame False {
                      n63 = local read "Samples per spot"() -> (w188:i32)
                      n64 = Greater?(x=w170, y=0) -> (0:w169:bool)
                      n65 = local read "slope"() -> (w179:i16)
                      n66 = case shown="真" w169 {
                        tunnel: [w195 w196] -> w173
                        tunnel: w172 -> [w195 w197]
                        frame False {
                        }
                        frame True {
                          n67 = local read "first"() -> (w198:dbl)
                          n68 = Add(x=w198, y=w197) -> (x+y=w196:dbl)
                        }
                      }
                      n69 = Subtract(x=w188, y=0) -> (x-y=w194:i32)
                      n70 = local read "dwell time"() -> (w178:i16)
                      n71 = Subtract(x=w188, y=w179) -> (x-y=w189:i32)
                      n72 = Multiply(x=w188, y=w186) -> (x*y=w191:i32)
                      n73 = for {
                        N: w194 -> [_]
                        tunnel: w191 -> [w291]
                        shift-right: [w290] -> w183
                        shift-left: w184 -> [w289]
                        tunnel: w175 -> [w285]
                        i -> [w288]
                        n74 = Less?(x=w288, y=50) -> (x < y?=w286:bool)
                        n75 = case shown="真" w286 {
                          tunnel: w291 -> [_ w299]
                          tunnel: [w292 w298] -> w290
                          tunnel: w288 -> [_ w297]
                          tunnel: w289 -> [w292 w296]
                          tunnel: w285 -> [_ w293]
                          frame False {
                          }
                          frame True {
                            n76 = Add(x=w299, y=w297) -> (x+y=w294:i32)
                            n77 = Add(x=w293, y=w294) -> (x+y=w295:dbl)
                            n78 = Replace Array Subset(array=w296, new element=1.0 ("新元素/子数组"), index=w295) -> (w298:dbl[])
                          }
                        }
                      }
                      n79 = Subtract(x=w189, y=w178) -> (x-y=w180:i32)
                      n80 = for {
                        N: w180 -> [_]
                        tunnel: w173 -> [w314]
                        tunnel: w191 -> [w312]
                        shift-right: [w315] -> w192
                        shift-left: w187 -> [w316]
                        tunnel: w175 -> [w309]
                        i -> [w313]
                        n81 = Add(x=w312, y=w313) -> (x+y=w310:i32)
                        n82 = Add(x=w309, y=w310) -> (x+y=w311:dbl)
                        n83 = Replace Array Subset(array=w316, new element=w314, index=w311) -> (w315:dbl[])
                      }
                      n84 = for {
                        N: w180 -> [_]
                        tunnel: w176 -> [w306]
                        shift-right: [w307] -> w181
                        shift-left: w185 -> [w308]
                        tunnel: w191 -> [w304]
                        tunnel: w175 -> [w301]
                        i -> [w305]
                        n85 = Add(x=w304, y=w305) -> (x+y=w302:i32)
                        n86 = Add(x=w301, y=w302) -> (x+y=w303:dbl)
                        n87 = Replace Array Subset(array=w308, new element=w306, index=w303) -> (w307:dbl[])
                      }
                      n88 = Add(x=w180, y=w191) -> (x+y=w177:i32)
                      n89 = local read "Y size"() -> (w164:i32)
                      n90 = for {
                        N: w179 -> [_]
                        shift-right: [w283] -> w190
                        shift-left: w192 -> [w284]
                        tunnel: w173 -> [w271]
                        tunnel: w177 -> [w277]
                        tunnel: w175 -> [w274]
                        i -> [w278]
                        n91 = local read "slope"() -> (w280:i16)
                        n92 = Add(x=w277, y=w278) -> (x+y=w276:i32)
                        n93 = Add(x=1, y=w278) -> (x+y=w281:i32)
                        n94 = Divide(x=w271, y=w280) -> (x/y=w279:dbl)
                        n95 = Add(x=w274, y=w276) -> (x+y=w275:dbl)
                        n96 = Multiply(x=w279, y=w281) -> (x*y=w272:dbl)
                        n97 = Subtract(x=w271, y=w272) -> (x-y=w273:dbl)
                        n98 = Replace Array Subset(array=w284, new element=w273, index=w275) -> (w283:dbl[])
                      }
                      n99 = Subtract(x=w164, y=1) -> (x-y=w163:i32)
                      n100 = Less?(x=w182, y=w163) -> (x < y?=w168:bool)
                      n101 = Add(x=w179, y=w177) -> (x+y=w174:i32)
                      n102 = case shown="假" w168 {
                        tunnel: [w199 w235] -> w166
                        tunnel: w181 -> [w206 w237]
                        tunnel: w179 -> [w207 w239]
                        tunnel: w178 -> [w202 w238]
                        tunnel: w175 -> [w203 w234]
                        tunnel: w177 -> [w204 w233]
                        tunnel: w176 -> [w205 w230]
                        tunnel: w175 -> [w201 w232]
                        tunnel: w174 -> [w200 w231]
                        frame False {
                          n103 = for {
                            N: w207 -> [_]
                            shift-right: [w228] -> w208
                            shift-left: w206 -> [w229]
                            tunnel: w203 -> [w227]
                            tunnel: w204 -> [w226]
                            tunnel: w205 -> [w217]
                            i -> [w223]
                            n104 = Add(x=w226, y=w223) -> (x+y=w225:i32)
                            n105 = Increment(x=w223) -> (x+1=w221:i32)
                            n106 = local read "slope"() -> (w220:i16)
                            n107 = Add(x=w227, y=w225) -> (x+y=w224:dbl)
                            n108 = Divide(x=w217, y=w220) -> (x/y=w222:dbl)
                            n109 = Multiply(x=w222, y=w221) -> (x*y=w219:dbl)
                            n110 = Subtract(x=w217, y=w219) -> (x-y=w218:dbl)
                            n111 = Replace Array Subset(array=w229, new element=w218, index=w224) -> (w228:dbl[])
                          }
                          n112 = for {
                            N: w202 -> [_]
                            shift-right: [w215] -> w199
                            shift-left: w208 -> [w216]
                            tunnel: w201 -> [w213]
                            tunnel: w200 -> [w211]
                            i -> [w214]
                            n113 = Add(x=w211, y=w214) -> (x+y=w212:i32)
                            n114 = Add(x=w213, y=w212) -> (x+y=w210:dbl)
                            n115 = Replace Array Subset(array=w216, new element=0, index=w210) -> (w215:dbl[])
                          }
                        }
                        frame True {
                          n116 = for {
                            N: w239 -> [_]
                            shift-right: [w261] -> w236
                            shift-left: w237 -> [w262]
                            tunnel: w234 -> [w260]
                            tunnel: w233 -> [w259]
                            tunnel: w230 -> [w251]
                            i -> [w256]
                            n117 = Add(x=w259, y=w256) -> (x+y=w258:i32)
                            n118 = local read "slope"() -> (w249:i16)
                            n119 = Increment(x=w256) -> (x+1=w253:i32)
                            n120 = Add(x=w260, y=w258) -> (x+y=w257:dbl)
                            n121 = Divide(x=1, y=w249) -> (x/y=w254:dbl)
                            n122 = Multiply(x=w254, y=w253) -> (x*y=w252:dbl)
                            n123 = Add(x=w251, y=w252) -> (x+y=w250:dbl)
                            n124 = Replace Array Subset(array=w262, new element=w250, index=w257) -> (w261:dbl[])
                          }
                          n125 = for {
                            N: w238 -> [_]
                            shift-right: [w247] -> w235
                            shift-left: w236 -> [w248]
                            tunnel: w232 -> [w245]
                            tunnel: w231 -> [w243]
                            tunnel: w230 -> [w240]
                            i -> [w246]
                            n126 = Increment(x=w240) -> (x+1=w241:i32)
                            n127 = Add(x=w243, y=w246) -> (x+y=w244:i32)
                            n128 = Add(x=w245, y=w244) -> (x+y=w242:dbl)
                            n129 = Replace Array Subset(array=w248, new element=w241, index=w242) -> (w247:dbl[])
                          }
                        }
                      }
                      n130 = for {
                        N: w178 -> [_]
                        shift-right: [w269] -> w167
                        shift-left: w190 -> [w270]
                        tunnel: w174 -> [w267]
                        tunnel: w175 -> [w264]
                        i -> [w268]
                        n131 = Add(x=w267, y=w268) -> (x+y=w266:i32)
                        n132 = Add(x=w264, y=w266) -> (x+y=w265:dbl)
                        n133 = Replace Array Subset(array=w270, new element=0, index=w265) -> (w269:dbl[])
                      }
                    }
                    frame True {
                      n134 = local read "Samples per spot"() -> (w322:i32)
                      n135 = Greater?(x=w319, y=0) -> (0:w317:bool)
                      n136 = case shown="真" w317 {
                        tunnel: [w343 w345] -> w321
                        tunnel: w320 -> [w343 w346]
                        frame False {
                        }
                        frame True {
                          n137 = Add(x="first", y=w346) -> (x+y=w345:dbl)
                        }
                      }
                      n138 = Subtract(x=w322, y=0) -> (x-y=w336:i32)
                      n139 = Subtract(x=w322, y="slope") -> (x-y=w329:i32)
                      n140 = Multiply(x=w322, y=w338) -> (x*y=w332:i32)
                      n141 = for {
                        N: w336 -> [_]
                        tunnel: w332 -> [w392]
                        shift-right: [w391] -> w334
                        shift-left: w337 -> [w390]
                        tunnel: w323 -> [w386]
                        i -> [w389]
                        n142 = Less?(x=w389, y=50) -> (x < y?=w387:bool)
                        n143 = case shown="真" w387 {
                          tunnel: w392 -> [_ w400]
                          tunnel: [w393 w399] -> w391
                          tunnel: w389 -> [_ w398]
                          tunnel: w390 -> [w393 w397]
                          tunnel: w386 -> [_ w394]
                          frame False {
                          }
                          frame True {
                            n144 = Add(x=w400, y=w398) -> (x+y=w395:i32)
                            n145 = Add(x=w394, y=w395) -> (x+y=w396:dbl)
                            n146 = Replace Array Subset(array=w397, new element=1.0 ("新元素/子数组"), index=w396) -> (w399:dbl[])
                          }
                        }
                      }
                      n147 = Subtract(x=w329, y="dwell time") -> (x-y=w328:i32)
                      n148 = for {
                        N: w322 -> [_]
                        tunnel: w339 -> [w407]
                        shift-right: [w408] -> w340
                        shift-left: w341 -> [w409]
                        tunnel: w332 -> [w405]
                        tunnel: w323 -> [w402]
                        i -> [w406]
                        n149 = Add(x=w405, y=w406) -> (x+y=w403:i32)
                        n150 = Add(x=w402, y=w403) -> (x+y=w404:dbl)
                        n151 = Replace Array Subset(array=w409, new element=w407, index=w404) -> (w408:dbl[])
                      }
                      n152 = for {
                        N: w328 -> [_]
                        tunnel: w321 -> [w415]
                        tunnel: w332 -> [w413]
                        shift-right: [w416] -> w333
                        shift-left: w342 -> [w417]
                        tunnel: w323 -> [w410]
                        i -> [w414]
                        n153 = Add(x=w413, y=w414) -> (x+y=w411:i32)
                        n154 = Add(x=w410, y=w411) -> (x+y=w412:dbl)
                        n155 = Replace Array Subset(array=w417, new element=w415, index=w412) -> (w416:dbl[])
                      }
                      n156 = Add(x=w328, y=w332) -> (x+y=w324:i32)
                      n157 = for {
                        N: "slope" -> [_]
                        shift-right: [w380] -> w331
                        shift-left: w333 -> [w381]
                        tunnel: w321 -> [w374]
                        tunnel: w324 -> [w373]
                        tunnel: w323 -> [w370]
                        tunnel: w319 -> [w364]
                        i -> [w367]
                        n158 = local read "slope"() -> (w376:i16)
                        n159 = Add(x=w373, y=w367) -> (x+y=w372:i32)
                        n160 = Equal?(x=w364, y=0) -> (x = y?=w366:bool)
                        n161 = Add(x=1, y=w367) -> (x+y=w378:i32)
                        n162 = Add(x=w370, y=w372) -> (x+y=w371:dbl)
                        n163 = case shown="真" w366 {
                          tunnel: [1 w383] -> w368
                          frame False {
                          }
                          frame True {
                            n164 = local read "first"() -> (w385:dbl)
                            n165 = Add(x=1, y=w385) -> (x+y=w383:dbl)
                          }
                        }
                        n166 = Divide(x=w368, y=w376) -> (x/y=w375:dbl)
                        n167 = Multiply(x=w375, y=w378) -> (x*y=w369:dbl)
                        n168 = Add(x=w374, y=w369) -> (x+y=w377:dbl)
                        n169 = Replace Array Subset(array=w381, new element=w377, index=w371) -> (w380:dbl[])
                      }
                      n170 = Add(x="slope", y=w324) -> (x+y=w326:i32)
                      n171 = for {
                        N: "dwell time" -> [_]
                        shift-right: [w358] -> w330
                        shift-left: w331 -> [w359]
                        tunnel: w326 -> [w356]
                        tunnel: w321 -> [w355]
                        tunnel: w323 -> [w351]
                        tunnel: w319 -> [w349]
                        i -> [w357]
                        n172 = Equal?(x=w349, y=0) -> (x = y?=w348:bool)
                        n173 = case shown="真" w348 {
                          tunnel: [1 w361] -> w347
                          frame False {
                          }
                          frame True {
                            n174 = local read "first"() -> (w363:dbl)
                            n175 = Add(x=1, y=w363) -> (x+y=w361:dbl)
                          }
                        }
                        n176 = Add(x=w355, y=w347) -> (x+y=w354:dbl)
                        n177 = Add(x=w356, y=w357) -> (x+y=w353:i32)
                        n178 = Add(x=w351, y=w353) -> (x+y=w352:dbl)
                        n179 = Replace Array Subset(array=w359, new element=w354, index=w352) -> (w358:dbl[])
                      }
                    }
                  }
                }
              }
            }
          }
          n180 = for {
            N: w60 -> [_]
            shift-right: [w75] -> w61
            shift-left: w62 -> [w76]
            tunnel: w59 -> [w74]
            tunnel: w56 -> [w71]
            i -> [w73]
            n181 = Add(x=w71, y=w73) -> (x+y=w72:dbl)
            n182 = Replace Array Subset(array=w76, new element=w74, index=w72) -> (w75:i32[])
          }
        }
      }
      "X index Array" <- w14
      "Y index Array" <- w13
      "Trigger" <- w12
      "nanoZ" <- w15
      "DO" <- w5
      n183 = call "Convert to Dynamic Data3"("Array"=w12) -> ("Dynamic Data Type"=w20:dynamicdata)  [unwired: 3 in]
      n184 = call "Convert to Dynamic Data"("Array"=w14) -> ("Dynamic Data Type"=w35:dynamicdata)  [unwired: 3 in]
      n185 = call "Convert to Dynamic Data2"("Array"=w13) -> ("Dynamic Data Type"=w34:dynamicdata)  [unwired: 3 in]
      n186 = call "Convert to Dynamic Data4"("Array"=w15) -> ("Dynamic Data Type"=w19:dynamicdata)  [unwired: 3 in]
      n187 = Merge Signals(w35, w34, w20, w19) -> (→"Waveform Graph":dynamicdata)
    }
    frame #1 {
      n188 = local read "Trigger"() -> (w463:dbl[])
      n189 = local read "Y index Array"() -> (w469:dbl[])
      n190 = local read "X index Array"() -> (w470:dbl[])
      n191 = local read "scan range (um)"() -> (w462:dbl)
      n192 = local read "first"() -> (w451:dbl)
      n193 = Multiply(x=w463, y="AmplitudeC") -> (x*y=w443:dbl[])
      "Trigger output" <- w443
      n194 = local read "nanoZ"() -> (w460:dbl[])
      n195 = Divide(x=w462, y=2) -> (x/y=w459:dbl)
      n196 = Multiply(x=w459, y=0.025) -> (x*y=w457:dbl)
      n197 = Subtract(x=w460, y=w457) -> (x-y=w447:dbl[])
      n198 = local read "X Size"() -> (w448:i32)
      n199 = Multiply(x="calibration", y=0.025) -> (x*y=w444:dbl)
      n200 = Subtract(x=w447, y=w444) -> (x-y=w426:dbl[])
      n201 = Add(x=w426, y=5) -> (x+y=w424:dbl[])
      "nanoZ output" <- w424
      n202 = Decrement(x=w448) -> (x-1=w449:i32)
      n203 = Divide(x="AmplitudeX", y=w449) -> (x/y=w455:dbl)
      n204 = Add(x=w449, y=w451) -> (x+y=w454:dbl)
      n205 = Multiply(x=w455, y=w454) -> (x*y=w452:dbl)
      n206 = local read "Y size"() -> (w441:i32)
      n207 = Add(x=w449, y=w451) -> (x+y=w450:dbl)
      n208 = Decrement(x=w441) -> (x-1=w477:i32)
      n209 = Divide(x=w470, y=w450) -> (x/y=w481:dbl[])
      n210 = Divide(x=w469, y=w477) -> (x/y=w472:dbl[])
      n211 = Subtract(x=w481, y=0.5) -> (x-y=w479:dbl[])
      n212 = Subtract(x=w472, y=0.5) -> (x-y=w474:dbl[])
      n213 = Multiply(x=w479, y=2) -> (x*y=w478:dbl[])
      n214 = Multiply(x=w474, y="AmplitudeY") -> (x*y=w475:dbl[])
      n215 = Multiply(x=w478, y=w452) -> (x*y=w468:dbl[])
      n216 = Multiply(x=w475, y=2) -> (x*y=w466:dbl[])
      n217 = Subtract(x=w468, y="zero point") -> (x-y=w437:dbl[])
      n218 = Subtract(x=w466, y="zero point 2") -> (x-y=w428:dbl[])
      n219 = call <vilib>:"Smoothing Filter Coefficients.vi"("fs"=100, "time constant"=1, "half-width"=20) -> ("forward coefficients"=w434:dbl[], "reverse coefficients"=w435:dbl[])  [unwired: 6 in, 1 out]
      n220 = call <vilib>:"Smoothing Filter Coefficients.vi"("fs"=100, "time constant"=1, "half-width"=20) -> ("forward coefficients"=w429:dbl[], "reverse coefficients"=w430:dbl[])  [unwired: 6 in, 1 out]
      n221 = call-poly <vilib>:"Zero Phase Filter.vi"("Forward Coefficients"=w434, "Reverse Coefficients"=w435, "X"=w437) -> ("Filtered X"=w436:dbl[])  [unwired: 7 in, 1 out]
      "X output Array" <- w436
      n222 = call-poly <vilib>:"Zero Phase Filter.vi"("Forward Coefficients"=w429, "Reverse Coefficients"=w430, "X"=w428) -> ("Filtered X"=w427:dbl[])  [unwired: 7 in, 1 out]
      "Y output Array" <- w427
      n223 = Build Array "Array creation"(w436, w427, w443, w424) -> (→"AO Data":dbl[][])
    }
    frame #2 {
      n224 = local read "Trigger output"() -> (w489:dbl[])
      n225 = local read "X output Array"() -> (w491:dbl[])
      n226 = local read "nanoZ output"() -> (w483:dbl[])
      n227 = local read "Y output Array"() -> (w492:dbl[])
      n228 = call <vilib>:"GetDateTimeInSecsCompatVI.vi"() -> ("double precision float"=w493:dbl)  [unwired: 1 in]
      "time" <- w493
      n229 = To Time Stamp(1:w493) -> (0:w484:timestamp)
      n230 = Bundle By Name("t0"=w484, "dt"="dt", "Y"=w491) -> (w488:waveform(dbl))  [unwired: 1 in]
      n231 = Bundle By Name("t0"=w484, "dt"="dt", "Y"=w492) -> (w487:waveform(dbl))  [unwired: 1 in]
      n232 = Bundle By Name("t0"=w484, "dt"="dt", "Y"=w489) -> (w486:waveform(dbl))  [unwired: 1 in]
      n233 = Bundle By Name("t0"=w484, "dt"="dt", "Y"=w483) -> (w482:waveform(dbl))  [unwired: 1 in]
      n234 = Build Array(w488, w487, w486, w482) -> (→"Output Graph" →"XY Scan":waveform(dbl)[])
    }
  }
